vi "Set_Source_RESTfulVI_Data.vi"(8 "error in (no error)":errorcluster, 10 "RESTful VI configuration":T1={"Service VI Type"=enum."Web Method", "Load VI at statup"=TRUE, "Keep VI in memory"=TRUE, "Output type"=enum."Terminal", "Output format"=enum."XML", "Use headers"=TRUE, "Buffered"=TRUE, "eng_Load VI by name"=FALSE}, 11 "Class in":refnum<class "AB_Source_RESTfulVI.lvclass">) -> (0 "error out":errorcluster, 3 "Class out":refnum<class "AB_Source_RESTfulVI.lvclass">)   [LabVIEW 2020, in "AB_Source_RESTfulVI.lvclass"]
uses:
  <vilib>/AppBuilder/AB_Classes/Source/RESTfulVI/AB_Source_RESTfulVI.lvclass
  <vilib>/AppBuilder/AB_Classes/Source/RESTfulVI/Configure_RESTfulVI/AB_RESTful_Configuration.ctl
  <vilib>/AppBuilder/AB_Classes/Source/RESTfulVI/Configure_RESTfulVI/AB_RESTful_VIType.ctl
  <vilib>/AppBuilder/AB_Classes/Source/RESTfulVI/Configure_RESTfulVI/AB_RESTful_OutputType.ctl
  <vilib>/AppBuilder/AB_Classes/Source/RESTfulVI/Configure_RESTfulVI/AB_RESTful_OutputFormat.ctl
  <vilib>/AppBuilder/AB_Classes/Source/RESTfulVI/AB_Source_RESTfulVI.lvclass/AB_Source_RESTfulVI.ctl
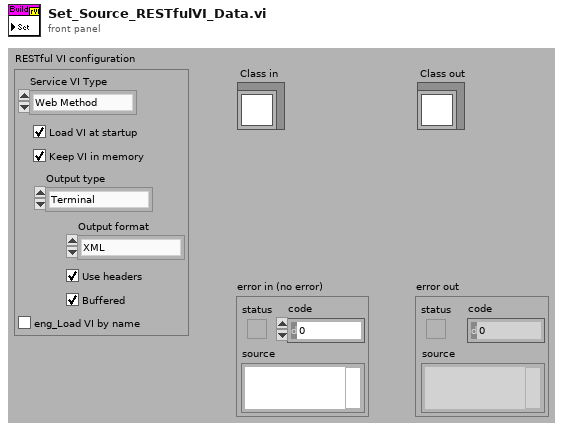
[diagram p1: front panel]
types:
  T1 = typedef "AB_RESTful_Configuration.ctl" = cluster{"Service VI Type":T2, "Load VI at statup":bool, "Keep VI in memory":bool, "Output type":T3, "Output format":T4, "Use headers":bool, "Buffered":bool, "eng_Load VI by name":bool}
  T2 = typedef "AB_RESTful_VIType.ctl" = enum32{"Web Method", "Auxiliary", "eng_Internal", "eng_Content"}
  T3 = typedef "AB_RESTful_OutputType.ctl" = enum32{"Terminal", "Stream"}
  T4 = typedef "AB_RESTful_OutputFormat.ctl" = enum32{"XML", "Text", "HTML", "JSON"}
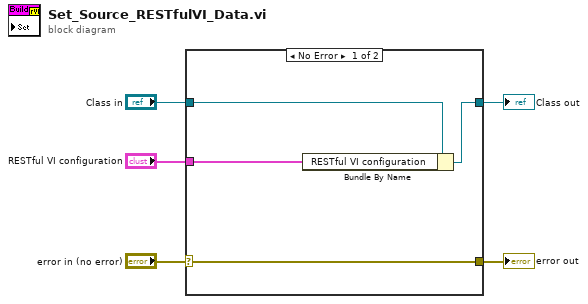
[diagram p0: block diagram]
diagram:
  n1 = case shown="No Error" "error in (no error)" {
    selector: "error in (no error)" -> [w9 w11]
    tunnel: [w9 w11] -> w4
    tunnel: "Class in" -> [w8 w10]
    tunnel: [w7 w10] -> w2
    tunnel: "RESTful VI configuration" -> [w6 _]
    frame No Error {
      n2 = Bundle By Name(cluster=w8, "RESTful VI configuration"=w6) -> (w7:refnum<class "AB_Source_RESTfulVI.lvclass">)
    }
    frame Error {
    }
  }
  "error out" <- w4
  "Class out" <- w2
